vi "ProfilerTest.vi"() -> ()   [LabVIEW 2014] (continued)
"delVelocity"=0.0}, {"Time"=36.65000000000128, "delVelocity"=0.0}, {"Time"=36.660000000001276, "delVelocity"=0.0}, {"Time"=36.670000000001274, "delVelocity"=0.0}, {"Time"=36.68000000000127, "delVelocity"=0.0}, {"Time"=36.69000000000127, "delVelocity"=0.0}, {"Time"=36.70000000000127, "delVelocity"=0.0}, {"Time"=36.710000000001266, "delVelocity"=0.0}, {"Time"=36.720000000001264, "delVelocity"=0.0}, {"Time"=36.73000000000126, "delVelocity"=0.0}, {"Time"=36.74000000000126, "delVelocity"=0.0}, {"Time"=36.75000000000126, "delVelocity"=0.0}, {"Time"=36.760000000001256, "delVelocity"=0.0}, {"Time"=36.770000000001254, "delVelocity"=0.0}, {"Time"=36.78000000000125, "delVelocity"=0.0}, {"Time"=36.79000000000125, "delVelocity"=0.0}, {"Time"=36.80000000000125, "delVelocity"=0.0}, {"Time"=36.810000000001246, "delVelocity"=0.0}, {"Time"=36.820000000001244, "delVelocity"=0.0}, {"Time"=36.83000000000124, "delVelocity"=0.0}, {"Time"=36.84000000000124, "delVelocity"=0.0}, {"Time"=36.85000000000124, "delVelocity"=0.0}, {"Time"=36.860000000001236, "delVelocity"=0.0}, {"Time"=36.870000000001234, "delVelocity"=0.0}, {"Time"=36.88000000000123, "delVelocity"=0.0}, {"Time"=36.89000000000123, "delVelocity"=0.0}, {"Time"=36.90000000000123, "delVelocity"=0.0}, {"Time"=36.910000000001226, "delVelocity"=0.0}, {"Time"=36.920000000001224, "delVelocity"=0.0}, {"Time"=36.93000000000122, "delVelocity"=0.0}, {"Time"=36.94000000000122, "delVelocity"=0.0}, {"Time"=36.95000000000122, "delVelocity"=0.0}, {"Time"=36.960000000001216, "delVelocity"=0.0}, {"Time"=36.970000000001214, "delVelocity"=0.0}, {"Time"=36.98000000000121, "delVelocity"=0.0}, {"Time"=36.99000000000121, "delVelocity"=0.0}, {"Time"=37.00000000000121, "delVelocity"=0.0}, {"Time"=37.010000000001206, "delVelocity"=0.0}, {"Time"=37.020000000001204, "delVelocity"=0.0}, {"Time"=37.0300000000012, "delVelocity"=0.0}, {"Time"=37.0400000000012, "delVelocity"=0.0}, {"Time"=37.0500000000012, "delVelocity"=0.0}, {"Time"=37.060000000001196, "delVelocity"=0.0}, {"Time"=37.070000000001194, "delVelocity"=0.0}, {"Time"=37.08000000000119, "delVelocity"=0.0}, {"Time"=37.09000000000119, "delVelocity"=0.0}, {"Time"=37.10000000000119, "delVelocity"=0.0}, {"Time"=37.110000000001186, "delVelocity"=0.0}, {"Time"=37.120000000001184, "delVelocity"=0.0}, {"Time"=37.13000000000118, "delVelocity"=0.0}, {"Time"=37.14000000000118, "delVelocity"=0.0}, {"Time"=37.15000000000118, "delVelocity"=0.0}, {"Time"=37.160000000001176, "delVelocity"=0.0}, {"Time"=37.170000000001174, "delVelocity"=0.0}, {"Time"=37.18000000000117, "delVelocity"=0.0}, {"Time"=37.19000000000117, "delVelocity"=0.0}, {"Time"=37.20000000000117, "delVelocity"=0.0}, {"Time"=37.210000000001166, "delVelocity"=0.0}, {"Time"=37.220000000001164, "delVelocity"=0.0}, {"Time"=37.23000000000116, "delVelocity"=0.0}, {"Time"=37.24000000000116, "delVelocity"=0.0}, {"Time"=37.25000000000116, "delVelocity"=0.0}, {"Time"=37.260000000001156, "delVelocity"=0.0}, {"Time"=37.270000000001154, "delVelocity"=0.0}, {"Time"=37.28000000000115, "delVelocity"=0.0}, {"Time"=37.29000000000115, "delVelocity"=0.0}, {"Time"=37.30000000000115, "delVelocity"=0.0}, {"Time"=37.310000000001146, "delVelocity"=0.0}, {"Time"=37.320000000001144, "delVelocity"=0.0}, {"Time"=37.33000000000114, "delVelocity"=0.0}, {"Time"=37.34000000000114, "delVelocity"=0.0}, {"Time"=37.35000000000114, "delVelocity"=0.0}, {"Time"=37.360000000001136, "delVelocity"=0.0}, {"Time"=37.370000000001134, "delVelocity"=0.0}, {"Time"=37.38000000000113, "delVelocity"=0.0}, {"Time"=37.39000000000113, "delVelocity"=0.0}, {"Time"=37.40000000000113, "delVelocity"=0.0}, {"Time"=37.410000000001126, "delVelocity"=0.0}, {"Time"=37.420000000001124, "delVelocity"=0.0}, {"Time"=37.43000000000112, "delVelocity"=0.0}, {"Time"=37.44000000000112, "delVelocity"=0.0}, {"Time"=37.45000000000112, "delVelocity"=0.0}, {"Time"=37.460000000001116, "delVelocity"=0.0}, {"Time"=37.470000000001114, "delVelocity"=0.0}, {"Time"=37.48000000000111, "delVelocity"=0.0}, {"Time"=37.49000000000111, "delVelocity"=0.0}, {"Time"=37.50000000000111, "delVelocity"=0.0}, {"Time"=37.51000000000111, "delVelocity"=0.0}, {"Time"=37.520000000001104, "delVelocity"=0.0}, {"Time"=37.5300000000011, "delVelocity"=0.0}, {"Time"=37.5400000000011, "delVelocity"=0.0}, {"Time"=37.5500000000011, "delVelocity"=0.0}, {"Time"=37.5600000000011, "delVelocity"=0.0}, {"Time"=37.570000000001095, "delVelocity"=0.0}, {"Time"=37.58000000000109, "delVelocity"=0.0}, {"Time"=37.59000000000109, "delVelocity"=0.0}, {"Time"=37.60000000000109, "delVelocity"=0.0}, {"Time"=37.61000000000109, "delVelocity"=0.0}, {"Time"=37.620000000001085, "delVelocity"=0.0}, {"Time"=37.63000000000108, "delVelocity"=0.0}, {"Time"=37.64000000000108, "delVelocity"=0.0}, {"Time"=37.65000000000108, "delVelocity"=0.0}, {"Time"=37.66000000000108, "delVelocity"=0.0}, {"Time"=37.670000000001075, "delVelocity"=0.0}, {"Time"=37.68000000000107, "delVelocity"=0.0}, {"Time"=37.69000000000107, "delVelocity"=0.0}, {"Time"=37.70000000000107, "delVelocity"=0.0}, {"Time"=37.71000000000107, "delVelocity"=0.0}, {"Time"=37.720000000001065, "delVelocity"=0.0}, {"Time"=37.73000000000106, "delVelocity"=0.0}, {"Time"=37.74000000000106, "delVelocity"=0.0}, {"Time"=37.75000000000106, "delVelocity"=0.0}, {"Time"=37.76000000000106, "delVelocity"=0.0}, {"Time"=37.770000000001055, "delVelocity"=0.0}, {"Time"=37.78000000000105, "delVelocity"=0.0}, {"Time"=37.79000000000105, "delVelocity"=0.0}, {"Time"=37.80000000000105, "delVelocity"=0.0}, {"Time"=37.81000000000105, "delVelocity"=0.0}, {"Time"=37.820000000001045, "delVelocity"=0.0}, {"Time"=37.83000000000104, "delVelocity"=0.0}, {"Time"=37.84000000000104, "delVelocity"=0.0}, {"Time"=37.85000000000104, "delVelocity"=0.0}, {"Time"=37.86000000000104, "delVelocity"=0.0}, {"Time"=37.870000000001035, "delVelocity"=0.0}, {"Time"=37.88000000000103, "delVelocity"=0.0}, {"Time"=37.89000000000103, "delVelocity"=0.0}, {"Time"=37.90000000000103, "delVelocity"=0.0}, {"Time"=37.91000000000103, "delVelocity"=0.0}, {"Time"=37.920000000001025, "delVelocity"=0.0}, {"Time"=37.93000000000102, "delVelocity"=0.0}, {"Time"=37.94000000000102, "delVelocity"=0.0}, {"Time"=37.95000000000102, "delVelocity"=0.0}, {"Time"=37.96000000000102, "delVelocity"=0.0}, {"Time"=37.970000000001015, "delVelocity"=0.0}, {"Time"=37.98000000000101, "delVelocity"=0.0}, {"Time"=37.99000000000101, "delVelocity"=0.0}, {"Time"=38.00000000000101, "delVelocity"=0.0}, {"Time"=38.01000000000101, "delVelocity"=0.0}, {"Time"=38.020000000001005, "delVelocity"=0.0}, {"Time"=38.030000000001, "delVelocity"=0.0}, {"Time"=38.040000000001, "delVelocity"=0.0}, {"Time"=38.050000000001, "delVelocity"=0.0}, {"Time"=38.060000000001, "delVelocity"=0.0}, {"Time"=38.070000000000995, "delVelocity"=0.0}, {"Time"=38.08000000000099, "delVelocity"=0.0}, {"Time"=38.09000000000099, "delVelocity"=0.0}, {"Time"=38.10000000000099, "delVelocity"=0.0}, {"Time"=38.11000000000099, "delVelocity"=0.0}, {"Time"=38.120000000000985, "delVelocity"=0.0}, {"Time"=38.13000000000098, "delVelocity"=0.0}, {"Time"=38.14000000000098, "delVelocity"=0.0}, {"Time"=38.15000000000098, "delVelocity"=0.0}, {"Time"=38.16000000000098, "delVelocity"=0.0}, {"Time"=38.170000000000975, "delVelocity"=0.0}, {"Time"=38.18000000000097, "delVelocity"=0.0}, {"Time"=38.19000000000097, "delVelocity"=0.0}, {"Time"=38.20000000000097, "delVelocity"=0.0}, {"Time"=38.21000000000097, "delVelocity"=0.0}, {"Time"=38.220000000000965, "delVelocity"=0.0}, {"Time"=38.23000000000096, "delVelocity"=0.0}, {"Time"=38.24000000000096, "delVelocity"=0.0}, {"Time"=38.25000000000096, "delVelocity"=0.0}, {"Time"=38.26000000000096, "delVelocity"=0.0}, {"Time"=38.270000000000955, "delVelocity"=0.0}, {"Time"=38.28000000000095, "delVelocity"=0.0}, {"Time"=38.29000000000095, "delVelocity"=0.0}, {"Time"=38.30000000000095, "delVelocity"=0.0}, {"Time"=38.31000000000095, "delVelocity"=0.0}, {"Time"=38.320000000000945, "delVelocity"=0.0}, {"Time"=38.33000000000094, "delVelocity"=0.0}, {"Time"=38.34000000000094, "delVelocity"=0.0}, {"Time"=38.35000000000094, "delVelocity"=0.0}, {"Time"=38.36000000000094, "delVelocity"=0.0}, {"Time"=38.370000000000935, "delVelocity"=0.0}, {"Time"=38.38000000000093, "delVelocity"=0.0}, {"Time"=38.39000000000093, "delVelocity"=0.0}, {"Time"=38.40000000000093, "delVelocity"=0.0}, {"Time"=38.41000000000093, "delVelocity"=0.0}, {"Time"=38.420000000000925, "delVelocity"=0.0}, {"Time"=38.43000000000092, "delVelocity"=0.0}, {"Time"=38.44000000000092, "delVelocity"=0.0}, {"Time"=38.45000000000092, "delVelocity"=0.0}, {"Time"=38.46000000000092, "delVelocity"=0.0}, {"Time"=38.470000000000915, "delVelocity"=0.0}, {"Time"=38.48000000000091, "delVelocity"=0.0}, {"Time"=38.49000000000091, "delVelocity"=0.0}, {"Time"=38.50000000000091, "delVelocity"=0.0}, {"Time"=38.51000000000091, "delVelocity"=0.0}, {"Time"=38.520000000000906, "delVelocity"=0.0}, {"Time"=38.5300000000009, "delVelocity"=0.0}, {"Time"=38.5400000000009, "delVelocity"=0.0}, {"Time"=38.5500000000009, "delVelocity"=0.0}, {"Time"=38.5600000000009, "delVelocity"=0.0}, {"Time"=38.570000000000896, "delVelocity"=0.0}, {"Time"=38.580000000000894, "delVelocity"=0.0}, {"Time"=38.59000000000089, "delVelocity"=0.0}, {"Time"=38.60000000000089, "delVelocity"=0.0}, {"Time"=38.61000000000089, "delVelocity"=0.0}, {"Time"=38.620000000000886, "delVelocity"=0.0}, {"Time"=38.630000000000884, "delVelocity"=0.0}, {"Time"=38.64000000000088, "delVelocity"=0.0}, {"Time"=38.65000000000088, "delVelocity"=0.0}, {"Time"=38.66000000000088, "delVelocity"=0.0}, {"Time"=38.670000000000876, "delVelocity"=0.0}, {"Time"=38.680000000000874, "delVelocity"=0.0}, {"Time"=38.69000000000087, "delVelocity"=0.0}, {"Time"=38.70000000000087, "delVelocity"=0.0}, {"Time"=38.71000000000087, "delVelocity"=0.0}, {"Time"=38.720000000000866, "delVelocity"=0.0}, {"Time"=38.730000000000864, "delVelocity"=0.0}, {"Time"=38.74000000000086, "delVelocity"=0.0}, {"Time"=38.75000000000086, "delVelocity"=0.0}, {"Time"=38.76000000000086, "delVelocity"=0.0}, {"Time"=38.770000000000856, "delVelocity"=0.0}, {"Time"=38.780000000000854, "delVelocity"=0.0}, {"Time"=38.79000000000085, "delVelocity"=0.0}, {"Time"=38.80000000000085, "delVelocity"=0.0}, {"Time"=38.81000000000085, "delVelocity"=0.0}, {"Time"=38.820000000000846, "delVelocity"=0.0}, {"Time"=38.830000000000844, "delVelocity"=0.0}, {"Time"=38.84000000000084, "delVelocity"=0.0}, {"Time"=38.85000000000084, "delVelocity"=0.0}, {"Time"=38.86000000000084, "delVelocity"=0.0}, {"Time"=38.870000000000836, "delVelocity"=0.0}, {"Time"=38.880000000000834, "delVelocity"=0.0}, {"Time"=38.89000000000083, "delVelocity"=0.0}, {"Time"=38.90000000000083, "delVelocity"=0.0}, {"Time"=38.91000000000083, "delVelocity"=0.0}, {"Time"=38.920000000000826, "delVelocity"=0.0}, {"Time"=38.930000000000824, "delVelocity"=0.0}, {"Time"=38.94000000000082, "delVelocity"=0.0}, {"Time"=38.95000000000082, "delVelocity"=0.0}, {"Time"=38.96000000000082, "delVelocity"=0.0}, {"Time"=38.970000000000816, "delVelocity"=0.0}, {"Time"=38.980000000000814, "delVelocity"=0.0}, {"Time"=38.99000000000081, "delVelocity"=0.0}, {"Time"=39.00000000000081, "delVelocity"=0.0}, {"Time"=39.01000000000081, "delVelocity"=0.0}, {"Time"=39.020000000000806, "delVelocity"=0.0}, {"Time"=39.030000000000804, "delVelocity"=0.0}, {"Time"=39.0400000000008, "delVelocity"=0.0}, {"Time"=39.0500000000008, "delVelocity"=0.0}, {"Time"=39.0600000000008, "delVelocity"=0.0}, {"Time"=39.070000000000796, "delVelocity"=0.0}, {"Time"=39.080000000000794, "delVelocity"=0.0}, {"Time"=39.09000000000079, "delVelocity"=0.0}, {"Time"=39.10000000000079, "delVelocity"=0.0}, {"Time"=39.11000000000079, "delVelocity"=0.0}, {"Time"=39.120000000000786, "delVelocity"=0.0}, {"Time"=39.130000000000784, "delVelocity"=0.0}, {"Time"=39.14000000000078, "delVelocity"=0.0}, {"Time"=39.15000000000078, "delVelocity"=0.0}, {"Time"=39.16000000000078, "delVelocity"=0.0}, {"Time"=39.170000000000776, "delVelocity"=0.0}, {"Time"=39.180000000000774, "delVelocity"=0.0}, {"Time"=39.19000000000077, "delVelocity"=0.0}, {"Time"=39.20000000000077, "delVelocity"=0.0}, {"Time"=39.21000000000077, "delVelocity"=0.0}, {"Time"=39.220000000000766, "delVelocity"=0.0}, {"Time"=39.230000000000764, "delVelocity"=0.0}, {"Time"=39.24000000000076, "delVelocity"=0.0}, {"Time"=39.25000000000076, "delVelocity"=0.0}, {"Time"=39.26000000000076, "delVelocity"=0.0}, {"Time"=39.270000000000756, "delVelocity"=0.0}, {"Time"=39.280000000000754, "delVelocity"=0.0}, {"Time"=39.29000000000075, "delVelocity"=0.0}, {"Time"=39.30000000000075, "delVelocity"=0.0}, {"Time"=39.31000000000075, "delVelocity"=0.0}, {"Time"=39.320000000000746, "delVelocity"=0.0}, {"Time"=39.330000000000744, "delVelocity"=0.0}, {"Time"=39.34000000000074, "delVelocity"=0.0}, {"Time"=39.35000000000074, "delVelocity"=0.0}, {"Time"=39.36000000000074, "delVelocity"=0.0}, {"Time"=39.370000000000736, "delVelocity"=0.0}, {"Time"=39.380000000000734, "delVelocity"=0.0}, {"Time"=39.39000000000073, "delVelocity"=0.0}, {"Time"=39.40000000000073, "delVelocity"=0.0}, {"Time"=39.41000000000073, "delVelocity"=0.0}, {"Time"=39.42000000000073, "delVelocity"=0.0}, {"Time"=39.430000000000724, "delVelocity"=0.0}, {"Time"=39.44000000000072, "delVelocity"=0.0}, {"Time"=39.45000000000072, "delVelocity"=0.0}, {"Time"=39.46000000000072, "delVelocity"=0.0}, {"Time"=39.47000000000072, "delVelocity"=0.0}, {"Time"=39.480000000000715, "delVelocity"=0.0}, {"Time"=39.49000000000071, "delVelocity"=0.0}, {"Time"=39.50000000000071, "delVelocity"=0.0}, {"Time"=39.51000000000071, "delVelocity"=0.0}, {"Time"=39.52000000000071, "delVelocity"=0.0}, {"Time"=39.530000000000705, "delVelocity"=0.0}, {"Time"=39.5400000000007, "delVelocity"=0.0}, {"Time"=39.5500000000007, "delVelocity"=0.0}, {"Time"=39.5600000000007, "delVelocity"=0.0}, {"Time"=39.5700000000007, "delVelocity"=0.0}, {"Time"=39.580000000000695, "delVelocity"=0.0}, {"Time"=39.59000000000069, "delVelocity"=0.0}, {"Time"=39.60000000000069, "delVelocity"=0.0}, {"Time"=39.61000000000069, "delVelocity"=0.0}, {"Time"=39.62000000000069, "delVelocity"=0.0}, {"Time"=39.630000000000685, "delVelocity"=0.0}, {"Time"=39.64000000000068, "delVelocity"=0.0}, {"Time"=39.65000000000068, "delVelocity"=0.0}, {"Time"=39.66000000000068, "delVelocity"=0.0}, {"Time"=39.67000000000068, "delVelocity"=0.0}, {"Time"=39.680000000000675, "delVelocity"=0.0}, {"Time"=39.69000000000067, "delVelocity"=0.0}, {"Time"=39.70000000000067, "delVelocity"=0.0}, {"Time"=39.71000000000067, "delVelocity"=0.0}, {"Time"=39.72000000000067, "delVelocity"=0.0}, {"Time"=39.730000000000665, "delVelocity"=0.0}, {"Time"=39.74000000000066, "delVelocity"=0.0}, {"Time"=39.75000000000066, "delVelocity"=0.0}, {"Time"=39.76000000000066, "delVelocity"=0.0}, {"Time"=39.77000000000066, "delVelocity"=0.0}, {"Time"=39.780000000000655, "delVelocity"=0.0}, {"Time"=39.79000000000065, "delVelocity"=0.0}, {"Time"=39.80000000000065, "delVelocity"=0.0}, {"Time"=39.81000000000065, "delVelocity"=0.0}, {"Time"=39.82000000000065, "delVelocity"=0.0}, {"Time"=39.830000000000645, "delVelocity"=0.0}, {"Time"=39.84000000000064, "delVelocity"=0.0}, {"Time"=39.85000000000064, "delVelocity"=0.0}, {"Time"=39.86000000000064, "delVelocity"=0.0}, {"Time"=39.87000000000064, "delVelocity"=0.0}, {"Time"=39.880000000000635, "delVelocity"=0.0}, {"Time"=39.89000000000063, "delVelocity"=0.0}, {"Time"=39.90000000000063, "delVelocity"=0.0}, {"Time"=39.91000000000063, "delVelocity"=0.0}, {"Time"=39.92000000000063, "delVelocity"=0.0}, {"Time"=39.930000000000625, "delVelocity"=0.0}, {"Time"=39.94000000000062, "delVelocity"=0.0}, {"Time"=39.95000000000062, "delVelocity"=0.0}, {"Time"=39.96000000000062, "delVelocity"=0.0}, {"Time"=39.97000000000062, "delVelocity"=0.0}, {"Time"=39.980000000000615, "delVelocity"=0.0}, {"Time"=39.99000000000061, "delVelocity"=0.0}, {"Time"=0.0, "delVelocity"=0.0}]}, ...(4 in all)]
  out "yAccel":T4(array[cluster])=[{"A"=5.0, "B"=7.853981633974483, "Start"=-0.2, "End"=0.2, "Center"=0.0, "Velocity"=0.0, "Position"=0.0}, {"A"=-3.0533720235915274, "B"=16.375338351724178, "Start"=0.4040754888200826, "End"=0.5959245111799174, "Center"=0.5, "Velocity"=1.0, "Position"=0.4040754888200826}, {"A"=-5.0, "B"=5.553603672697958, "Start"=0.9242640687119285, "End"=1.4899494936611664, "Center"=1.2071067811865475, "Velocity"=0.7071067811865475, "Position"=0.8}, {"A"=0.0, "B"=0.0, "Start"=1.914213562373095, "End"=1.914213562373095, "Center"=1.914213562373095, "Velocity"=-0.7071067811865475, "Position"=0.5}, {"A"=5.0, "B"=5.553603672697958, "Start"=2.3384776310850235, "End"=2.9041630560342613, "Center"=2.6213203435596424, "Velocity"=-0.7071067811865475, "Position"=0.19999999999999998}, {"A"=-5.0, "B"=4.60075592255305, "Start"=2.9870057685088804, "End"=3.6698484809834993, "Center"=3.32842712474619, "Velocity"=0.7071067811865475, "Position"=0.2585786437626905}, {"A"=0.0, "B"=0.0, "Start"=3.82842712474619, "End"=3.82842712474619, "Center"=3.82842712474619, "Velocity"=-1.0, "Position"=0.0}]
  out "xAccel":T4(array[cluster])=[{"A"=0.0, "B"=0.0, "Start"=0.0, "End"=0.0, "Center"=0.0, "Velocity"=0.0, "Position"=0.0}, {"A"=4.7442499832879435, "B"=10.539073652554059, "Start"=0.35095499105709094, "End"=0.6490450089429091, "Center"=0.5, "Velocity"=0.0, "Position"=0.0}, {"A"=0.0, "B"=0.0, "Start"=1.2071067811865475, "End"=1.2071067811865475, "Center"=1.2071067811865475, "Velocity"=0.7071067811865475, "Position"=0.5}, {"A"=-5.0, "B"=5.553603672697958, "Start"=1.631370849898476, "End"=2.197056274847714, "Center"=1.914213562373095, "Velocity"=0.7071067811865475, "Position"=0.8}, {"A"=0.0, "B"=0.0, "Start"=2.6213203435596424, "End"=2.6213203435596424, "Center"=2.6213203435596424, "Velocity"=-0.7071067811865475, "Position"=0.5}, {"A"=4.7442499832879435, "B"=10.539073652554059, "Start"=3.1793821158032807, "End"=3.477472133689099, "Center"=3.32842712474619, "Velocity"=-0.7071067811865475, "Position"=0.10539073652554058}, {"A"=0.0, "B"=0.0, "Start"=3.82842712474619, "End"=3.82842712474619, "Center"=3.82842712474619, "Velocity"=0.0, "Position"=0.0}]
  out "Accel":cluster{cluster{"Time":dbl, "Velocity":dbl}[]}[](graph)=[{[{"Time"=0.0, "Velocity"=0.0}, {"Time"=0.0, "Velocity"=0.0}, {"Time"=0.0, "Velocity"=0.0}, {"Time"=0.0, "Velocity"=0.0}, {"Time"=0.0, "Velocity"=0.0}, {"Time"=0.0, "Velocity"=0.0}, {"Time"=0.0, "Velocity"=0.0}, {"Time"=0.0, "Velocity"=0.0}, {"Time"=0.0, "Velocity"=0.0}, {"Time"=0.0, "Velocity"=0.0}, {"Time"=0.0, "Velocity"=0.0}, {"Time"=0.0, "Velocity"=0.0}, {"Time"=0.0, "Velocity"=0.0}, {"Time"=0.0, "Velocity"=0.0}, {"Time"=0.0, "Velocity"=0.0}, {"Time"=0.0, "Velocity"=0.0}, {"Time"=0.0, "Velocity"=0.0}, {"Time"=0.0, "Velocity"=0.0}, {"Time"=0.0, "Velocity"=0.0}, {"Time"=0.0, "Velocity"=0.0}, {"Time"=0.0, "Velocity"=0.0}, {"Time"=0.0, "Velocity"=0.0}, {"Time"=0.0, "Velocity"=0.0}, {"Time"=0.0, "Velocity"=0.0}, {"Time"=0.0, "Velocity"=0.0}, {"Time"=0.0, "Velocity"=0.0}, {"Time"=0.0, "Velocity"=0.0}, {"Time"=0.0, "Velocity"=0.0}, {"Time"=0.0, "Velocity"=0.0}, {"Time"=0.0, "Velocity"=0.0}, {"Time"=0.0, "Velocity"=0.0}, {"Time"=0.0, "Velocity"=0.0}, {"Time"=0.0, "Velocity"=0.0}, {"Time"=0.0, "Velocity"=0.0}, {"Time"=0.0, "Velocity"=0.0}, {"Time"=0.0, "Velocity"=0.0}, {"Time"=0.0, "Velocity"=0.0}, {"Time"=0.0, "Velocity"=0.0}, {"Time"=0.0, "Velocity"=0.0}, {"Time"=0.0, "Velocity"=0.0}, {"Time"=0.0, "Velocity"=0.0}, {"Time"=0.0, "Velocity"=0.0}, {"Time"=0.0, "Velocity"=0.0}, {"Time"=0.0, "Velocity"=0.0}, {"Time"=0.0, "Velocity"=0.0}, {"Time"=0.0, "Velocity"=0.0}, {"Time"=0.0, "Velocity"=0.0}, {"Time"=0.0, "Velocity"=0.0}, {"Time"=0.0, "Velocity"=0.0}, {"Time"=0.0, "Velocity"=0.0}, {"Time"=0.0, "Velocity"=0.0}, {"Time"=0.0, "Velocity"=0.0}, {"Time"=0.0, "Velocity"=0.0}, {"Time"=0.0, "Velocity"=0.0}, {"Time"=0.0, "Velocity"=0.0}, {"Time"=0.0, "Velocity"=0.0}, {"Time"=0.0, "Velocity"=0.0}, {"Time"=0.0, "Velocity"=0.0}, {"Time"=0.0, "Velocity"=0.0}, {"Time"=0.0, "Velocity"=0.0}, {"Time"=0.0, "Velocity"=0.0}, {"Time"=0.0, "Velocity"=0.0}, {"Time"=0.0, "Velocity"=0.0}, {"Time"=0.0, "Velocity"=0.0}, {"Time"=0.0, "Velocity"=0.0}, {"Time"=0.0, "Velocity"=0.0}, {"Time"=0.0, "Velocity"=0.0}, {"Time"=0.0, "Velocity"=0.0}, {"Time"=0.0, "Velocity"=0.0}, {"Time"=0.0, "Velocity"=0.0}, {"Time"=0.0, "Velocity"=0.0}, {"Time"=0.0, "Velocity"=0.0}, {"Time"=0.0, "Velocity"=0.0}, {"Time"=0.0, "Velocity"=0.0}, {"Time"=0.0, "Velocity"=0.0}, {"Time"=0.0, "Velocity"=0.0}, {"Time"=0.0, "Velocity"=0.0}, {"Time"=0.0, "Velocity"=0.0}, {"Time"=0.0, "Velocity"=0.0}, {"Time"=0.0, "Velocity"=0.0}, {"Time"=0.0, "Velocity"=0.0}, {"Time"=0.0, "Velocity"=0.0}, {"Time"=0.0, "Velocity"=0.0}, {"Time"=0.0, "Velocity"=0.0}, {"Time"=0.0, "Velocity"=0.0}, {"Time"=0.0, "Velocity"=0.0}, {"Time"=0.0, "Velocity"=0.0}, {"Time"=0.0, "Velocity"=0.0}, {"Time"=0.0, "Velocity"=0.0}, {"Time"=0.0, "Velocity"=0.0}, {"Time"=0.0, "Velocity"=0.0}, {"Time"=0.0, "Velocity"=0.0}, {"Time"=0.0, "Velocity"=0.0}, {"Time"=0.0, "Velocity"=0.0}, {"Time"=0.0, "Velocity"=0.0}, {"Time"=0.0, "Velocity"=0.0}, {"Time"=0.0, "Velocity"=0.0}, {"Time"=0.0, "Velocity"=0.0}, {"Time"=0.0, "Velocity"=0.0}, {"Time"=0.0, "Velocity"=0.0}, {"Time"=0.0, "Velocity"=0.0}, {"Time"=0.35095531925568213, "Velocity"=5.50736024568391e-11}, {"Time"=0.3539359458930411, "Velocity"=0.004681003307826736}, {"Time"=0.3569169329724022, "Velocity"=0.018705771687410763}, {"Time"=0.3598980439615304, "Velocity"=0.04202011351167813}, {"Time"=0.3628788161034107, "Velocity"=0.07452740216306052}, {"Time"=0.3658595272222378, "Velocity"=0.11610053792080005}, {"Time"=0.3688406611141025, "Velocity"=0.16658382483664627}, {"Time"=0.3718215316238896, "Velocity"=0.2257671329984986}, {"Time"=0.37480228037519364, "Velocity"=0.29341803418359613}, {"Time"=0.3777830973771714, "Velocity"=0.3692736379683199}, {"Time"=0.380764072133267, "Velocity"=0.4530377768984485}, {"Time"=0.3837451854232035, "Velocity"=0.5443804709605526}, {"Time"=0.38672614678717, "Velocity"=0.642932269145972}, {"Time"=0.3897067735390129, "Velocity"=0.7482964854099229}, {"Time"=0.39268779230328543, "Velocity"=0.8600831387079992}, {"Time"=0.3956686493693256, "Velocity"=0.9778310646207633}, {"Time"=0.39864961030082646, "Velocity"=1.1010858577858063}, {"Time"=0.40163042391800347, "Velocity"=1.2293506118536994}, {"Time"=0.40461134537834614, "Velocity"=1.3621299917800744}, {"Time"=0.40759213500004476, "Velocity"=1.498889288710395}, {"Time"=0.4105733396656944, "Velocity"=1.6391143292638135}, {"Time"=0.4135539403558606, "Velocity"=1.7822035689878706}, {"Time"=0.4165348905749282, "Velocity"=1.9276376584907495}, {"Time"=0.41951578640723575, "Velocity"=2.0748232975591545}, {"Time"=0.42249679151073805, "Velocity"=2.223187700059486}, {"Time"=0.4254776474532113, "Velocity"=2.3721324733928784}, {"Time"=0.42845858580727364, "Velocity"=2.5210813296808565}, {"Time"=0.4314396484569505, "Velocity"=2.66944847406714}, {"Time"=0.4344202596314551, "Velocity"=2.816619916696366}, {"Time"=0.43740137519387107, "Velocity"=2.9620619079454316}, {"Time"=0.4403821725508091, "Velocity"=3.105160219697094}, {"Time"=0.44336302583933573, "Velocity"=3.245368375837273}, {"Time"=0.44634387547325305, "Velocity"=3.3821301821391057}, {"Time"=0.4493247970269584, "Velocity"=3.514909245469887}, {"Time"=0.45230571043094475, "Velocity"=3.6431778524652842}, {"Time"=0.4552867137489194, "Velocity"=3.766433786802063}, {"Time"=0.4582676835999003, "Velocity"=3.884185350994328}, {"Time"=0.46124842978267827, "Velocity"=3.99596107220399}, {"Time"=0.4642292839309622, "Velocity"=4.101332611153013}, {"Time"=0.46721035372627223, "Velocity"=4.199886840806099}, {"Time"=0.47019116678105355, "Velocity"=4.291219363025584}, {"Time"=0.47317195740077206, "Velocity"=4.37497793755458}, {"Time"=0.47615286456958295, "Velocity"=4.450835554257804}, {"Time"=0.479134006270323, "Velocity"=4.518494403973455}, {"Time"=0.48211476749612264, "Velocity"=4.577674138445382}, {"Time"=0.4850958093220748, "Velocity"=4.628154724183214}, {"Time"=0.48807652197732365, "Velocity"=4.669726851819185}, {"Time"=0.4910574291962836, "Velocity"=4.702234357339671}, {"Time"=0.4940382028607463, "Velocity"=4.725545104792937}, {"Time"=0.49701922558438005, "Velocity"=4.739569547693048}, {"Time"=0.5000002690275388, "Velocity"=4.744249999961862}, {"Time"=0.5029810686846331, "Velocity"=4.739568623821157}, {"Time"=0.5059620123716997, "Velocity"=4.725543755980428}, {"Time"=0.5089429652918902, "Velocity"=4.702230661326216}, {"Time"=0.5119236749950736, "Velocity"=4.669724402571721}, {"Time"=0.5149047704873164, "Velocity"=4.628145765646637}, {"Time"=0.5178856707272734, "Velocity"=4.577666072383549}, {"Time"=0.520866503859561, "Velocity"=4.518483543861212}, {"Time"=0.523847516316558, "Velocity"=4.450826379548527}, {"Time"=0.5268283322097902, "Velocity"=4.374970178476992}, {"Time"=0.5298090653014678, "Velocity"=4.291212542301367}, {"Time"=0.5327901478802014, "Velocity"=4.199870854007082}, {"Time"=0.5357708251342688, "Velocity"=4.101328878141011}, {"Time"=0.5387519365752801, "Velocity"=3.9959477190167645}, {"Time"=0.5417326532258172, "Velocity"=3.8841723745863823}, {"Time"=0.5447136608295621, "Velocity"=3.766418634790069}, {"Time"=0.5476947464554902, "Velocity"=3.6431585643356734}, {"Time"=0.5506753637730458, "Velocity"=3.514902199965208}, {"Time"=0.5536565483461207, "Velocity"=3.3821110079509995}, {"Time"=0.5566371342578786, "Velocity"=3.245360933108672}, {"Time"=0.5596181273960594, "Velocity"=3.1051459563777444}, {"Time"=0.5625990777602468, "Velocity"=2.9620399717640513}, {"Time"=0.5655800049566987, "Velocity"=2.8166069216136798}, {"Time"=0.568560732875166, "Velocity"=2.6694295578145515}, {"Time"=0.5715419247218683, "Velocity"=2.5210558535911827}, {"Time"=0.5745228056007107, "Velocity"=2.372109820695952}, {"Time"=0.5775037267700815, "Velocity"=2.223161837155251}, {"Time"=0.5804844515939579, "Velocity"=2.074811491335522}, {"Time"=0.5834654466221451, "Velocity"=1.9276210972758885}, {"Time"=0.5864463583362974, "Velocity"=1.782189103585959}, {"Time"=0.5894270243328484, "Velocity"=1.6390970200848998}, {"Time"=0.5924082186970084, "Velocity"=1.4988728457687575}, {"Time"=0.5953890228973194, "Velocity"=1.3621133304961972}, {"Time"=0.5983700078816026, "Velocity"=1.2293316924286313}, {"Time"=0.6013507854827487, "Velocity"=1.1010691492255635}, {"Time"=0.6043318079934541, "Velocity"=0.9778125639286918}, {"Time"=0.6073124405489622, "Velocity"=0.8600741679083297}, {"Time"=0.6102933319138173, "Velocity"=0.7482926418177279}, {"Time"=0.6132743316865582, "Velocity"=0.6429158922144192}, {"Time"=0.6162551894170679, "Velocity"=0.5443685243202626}, {"Time"=0.6192361682993021, "Velocity"=0.45303071077147344}, {"Time"=0.6222172382105677, "Velocity"=0.36926464717276025}, {"Time"=0.6251978283531981, "Velocity"=0.29341541516543757}, {"Time"=0.6281787093500688, "Velocity"=0.22576200288591172}, {"Time"=0.6311599266610616, "Velocity"=0.1665730061296175}, {"Time"=0.6341408500489021, "Velocity"=0.116094708820569}, {"Time"=0.6371216254044041, "Velocity"=0.07452191223685314}, {"Time"=0.6401025565856091, "Velocity"=0.042014486916333305}, {"Time"=0.6430832903776259, "Velocity"=0.0187043720224209}, {"Time"=0.6460641319394195, "Velocity"=0.004680758949891532}, {"Time"=0.6490452493606549, "Velocity"=3.1716017876300603e-11}, {"Time"=1.2071067811865475, "Velocity"=0.0}, {"Time"=1.2071067811865475, "Velocity"=0.0}, {"Time"=1.2071067811865475, "Velocity"=0.0}, {"Time"=1.2071067811865475, "Velocity"=0.0}, {"Time"=1.2071067811865475, "Velocity"=0.0}, {"Time"=1.2071067811865475, "Velocity"=0.0}, {"Time"=1.2071067811865475, "Velocity"=0.0}, {"Time"=1.2071067811865475, "Velocity"=0.0}, {"Time"=1.2071067811865475, "Velocity"=0.0}, {"Time"=1.2071067811865475, "Velocity"=0.0}, {"Time"=1.2071067811865475, "Velocity"=0.0}, {"Time"=1.2071067811865475, "Velocity"=0.0}, {"Time"=1.2071067811865475, "Velocity"=0.0}, {"Time"=1.2071067811865475, "Velocity"=0.0}, {"Time"=1.2071067811865475, "Velocity"=0.0}, {"Time"=1.2071067811865475, "Velocity"=0.0}, {"Time"=1.2071067811865475, "Velocity"=0.0}, {"Time"=1.2071067811865475, "Velocity"=0.0}, {"Time"=1.2071067811865475, "Velocity"=0.0}, {"Time"=1.2071067811865475, "Velocity"=0.0}, {"Time"=1.2071067811865475, "Velocity"=0.0}, {"Time"=1.2071067811865475, "Velocity"=0.0}, {"Time"=1.2071067811865475, "Velocity"=0.0}, {"Time"=1.2071067811865475, "Velocity"=0.0}, {"Time"=1.2071067811865475, "Velocity"=0.0}, {"Time"=1.2071067811865475, "Velocity"=0.0}, {"Time"=1.2071067811865475, "Velocity"=0.0}, {"Time"=1.2071067811865475, "Velocity"=0.0}, {"Time"=1.2071067811865475, "Velocity"=0.0}, {"Time"=1.2071067811865475, "Velocity"=0.0}, {"Time"=1.2071067811865475, "Velocity"=0.0}, {"Time"=1.2071067811865475, "Velocity"=0.0}, {"Time"=1.2071067811865475, "Velocity"=0.0}, {"Time"=1.2071067811865475, "Velocity"=0.0}, {"Time"=1.2071067811865475, "Velocity"=0.0}, {"Time"=1.2071067811865475, "Velocity"=0.0}, {"Time"=1.2071067811865475, "Velocity"=0.0}, {"Time"=1.2071067811865475, "Velocity"=0.0}, {"Time"=1.2071067811865475, "Velocity"=0.0}, {"Time"=1.2071067811865475, "Velocity"=0.0}, {"Time"=1.2071067811865475, "Velocity"=0.0}, {"Time"=1.2071067811865475, "Velocity"=0.0}, {"Time"=1.2071067811865475, "Velocity"=0.0}, {"Time"=1.2071067811865475, "Velocity"=0.0}, {"Time"=1.2071067811865475, "Velocity"=0.0}, {"Time"=1.2071067811865475, "Velocity"=0.0}, {"Time"=1.2071067811865475, "Velocity"=0.0}, {"Time"=1.2071067811865475, "Velocity"=0.0}, {"Time"=1.2071067811865475, "Velocity"=0.0}, {"Time"=1.2071067811865475, "Velocity"=0.0}, {"Time"=1.2071067811865475, "Velocity"=0.0}, {"Time"=1.2071067811865475, "Velocity"=0.0}, {"Time"=1.2071067811865475, "Velocity"=0.0}, {"Time"=1.2071067811865475, "Velocity"=0.0}, {"Time"=1.2071067811865475, "Velocity"=0.0}, {"Time"=1.2071067811865475, "Velocity"=0.0}, {"Time"=1.2071067811865475, "Velocity"=0.0}, {"Time"=1.2071067811865475, "Velocity"=0.0}, {"Time"=1.2071067811865475, "Velocity"=0.0}, {"Time"=1.2071067811865475, "Velocity"=0.0}, {"Time"=1.2071067811865475, "Velocity"=0.0}, {"Time"=1.2071067811865475, "Velocity"=0.0}, {"Time"=1.2071067811865475, "Velocity"=0.0}, {"Time"=1.2071067811865475, "Velocity"=0.0}, {"Time"=1.2071067811865475, "Velocity"=0.0}, {"Time"=1.2071067811865475, "Velocity"=0.0}, {"Time"=1.2071067811865475, "Velocity"=0.0}, {"Time"=1.2071067811865475, "Velocity"=0.0}, {"Time"=1.2071067811865475, "Velocity"=0.0}, {"Time"=1.2071067811865475, "Velocity"=0.0}, {"Time"=1.2071067811865475, "Velocity"=0.0}, {"Time"=1.2071067811865475, "Velocity"=0.0}, {"Time"=1.2071067811865475, "Velocity"=0.0}, {"Time"=1.2071067811865475, "Velocity"=0.0}, {"Time"=1.2071067811865475, "Velocity"=0.0}, {"Time"=1.2071067811865475, "Velocity"=0.0}, {"Time"=1.2071067811865475, "Velocity"=0.0}, {"Time"=1.2071067811865475, "Velocity"=0.0}, {"Time"=1.2071067811865475, "Velocity"=0.0}, {"Time"=1.2071067811865475, "Velocity"=0.0}, {"Time"=1.2071067811865475, "Velocity"=0.0}, {"Time"=1.2071067811865475, "Velocity"=0.0}, {"Time"=1.2071067811865475, "Velocity"=0.0}, {"Time"=1.2071067811865475, "Velocity"=0.0}, {"Time"=1.2071067811865475, "Velocity"=0.0}, {"Time"=1.2071067811865475, "Velocity"=0.0}, {"Time"=1.2071067811865475, "Velocity"=0.0}, {"Time"=1.2071067811865475, "Velocity"=0.0}, {"Time"=1.2071067811865475, "Velocity"=0.0}, {"Time"=1.2071067811865475, "Velocity"=0.0}, {"Time"=1.2071067811865475, "Velocity"=0.0}, {"Time"=1.2071067811865475, "Velocity"=0.0}, {"Time"=1.2071067811865475, "Velocity"=0.0}, {"Time"=1.2071067811865475, "Velocity"=0.0}, {"Time"=1.2071067811865475, "Velocity"=0.0}, {"Time"=1.2071067811865475, "Velocity"=0.0}, {"Time"=1.2071067811865475, "Velocity"=0.0}, {"Time"=1.2071067811865475, "Velocity"=0.0}, {"Time"=1.2071067811865475, "Velocity"=0.0}, {"Time"=1.2071067811865475, "Velocity"=0.0}, {"Time"=1.2071067811865475, "Velocity"=0.0}, {"Time"=1.6313709713857558, "Velocity"=-1.7080866399157617e-11}, {"Time"=1.6370282709806934, "Velocity"=-0.004933375727589114}, {"Time"=1.6426849079991253, "Velocity"=-0.019712884672038487}, {"Time"=1.6483415996983244, "Velocity"=-0.044280487862295104}, {"Time"=1.6539986753458422, "Velocity"=-0.07854178978642275}, {"Time"=1.6596556901806123, "Velocity"=-0.12235970811397348}, {"Time"=1.665312360236421, "Velocity"=-0.1755580957494901}, {"Time"=1.6709691529406534, "Velocity"=-0.23793084760329003}, {"Time"=1.676626212913127, "Velocity"=-0.30923433515789267}, {"Time"=1.6822827123498711, "Velocity"=-0.3891760634774344}, {"Time"=1.6879400617709552, "Velocity"=-0.47746107896069007}, {"Time"=1.6935962842751575, "Velocity"=-0.5737095830376884}, {"Time"=1.6992532063435852, "Velocity"=-0.6775718764786762}, {"Time"=1.7049105370471096, "Velocity"=-0.7886349059724539}, {"Time"=1.7105672640182004, "Velocity"=-0.9064401325634146}, {"Time"=1.7162236979713061, "Velocity"=-1.0305275471784532}, {"Time"=1.721880645195221, "Velocity"=-1.160425471206782}, {"Time"=1.7275375756120264, "Velocity"=-1.295609849283178}, {"Time"=1.733194266958434, "Velocity"=-1.4355415268732759}, {"Time"=1.7388511806477678, "Velocity"=-1.5796796348273192}, {"Time"=1.7445084006521792, "Velocity"=-1.7274579929979808}, {"Time"=1.7501651906164457, "Velocity"=-1.8782740498239738}, {"Time"=1.7558218830375498, "Velocity"=-2.031541058872726}, {"Time"=1.7614790199438888, "Velocity"=-2.1866690009673215}, {"Time"=1.7671359216104991, "Velocity"=-2.343027121799203}, {"Time"=1.7727927595404411, "Velocity"=-2.5000029834813993}, {"Time"=1.7784496560344534, "Velocity"=-2.6569804563884114}, {"Time"=1.7841064035118543, "Velocity"=-2.8133342845614884}, {"Time"=1.7897631395459257, "Velocity"=-2.9684512598511636}, {"Time"=1.7954199999975988, "Velocity"=-3.1217228953509206}, {"Time"=1.8010768994328874, "Velocity"=-3.272541898469922}, {"Time"=1.806733605263529, "Velocity"=-3.4203069841090854}, {"Time"=1.8123907523050318, "Velocity"=-3.5644513141656216}, {"Time"=1.818047178727535, "Velocity"=-3.7043767709226803}, {"Time"=1.8237041515421901, "Velocity"=-3.83956263130222}, {"Time"=1.8293612186562676, "Velocity"=-3.969463746218262}, {"Time"=1.8350181774083052, "Velocity"=-4.093562803594636}, {"Time"=1.8406747486420618, "Velocity"=-4.211364719437065}, {"Time"=1.8463318125129005, "Velocity"=-4.322422699677098}, {"Time"=1.851988715518848, "Velocity"=-4.4262850290876035}, {"Time"=1.8576453562736979, "Velocity"=-4.522540779260416}, {"Time"=1.8633022020871002, "Velocity"=-4.610818137383916}, {"Time"=1.8689592132708241, "Velocity"=-4.690767296734542}, {"Time"=1.8746157273145294, "Velocity"=-4.762064140129214}, {"Time"=1.8802727897096965, "Velocity"=-4.824440327506827}, {"Time"=1.8859296217848325, "Velocity"=-4.877640358565102}, {"Time"=1.8915865989596123, "Velocity"=-4.921458003809648}, {"Time"=1.8972436635459324, "Velocity"=-4.955719299066888}, {"Time"=1.9029002654742275, "Velocity"=-4.980286660385663}, {"Time"=1.9085572145244145, "Velocity"=-4.995066940400685}, {"Time"=1.9142142079681224, "Velocity"=-4.99999999999333}, {"Time"=1.919870458087822, "Velocity"=-4.995067511200252}, {"Time"=1.9255276604175486, "Velocity"=-4.980286918300999}, {"Time"=1.9311846920812694, "Velocity"=-4.95571744866967}, {"Time"=1.9368414152059714, "Velocity"=-4.92145790598746}, {"Time"=1.9424979698836047, "Velocity"=-4.877643862361085}, {"Time"=1.948154953909832, "Velocity"=-4.824442948248025}, {"Time"=1.9538121557145325, "Velocity"=-4.762065523089948}, {"Time"=1.9594690519357183, "Velocity"=-4.690763748968648}, {"Time"=1.9651252996623443, "Velocity"=-4.6108255507610725}, {"Time"=1.9707825265303958, "Velocity"=-4.522542692090294}, {"Time"=1.976439233805907, "Velocity"=-4.42628592603794}, {"Time"=1.982096169164168, "Velocity"=-4.322423047968585}, {"Time"=1.9877531161885007, "Velocity"=-4.2113674555412715}, {"Time"=1.9934097596440727, "Velocity"=-4.093564150396464}, {"Time"=1.999066384653616, "Velocity"=-3.969472657766189}, {"Time"=2.0047232700425024, "Velocity"=-3.839576192421264}, {"Time"=2.0103800975957924, "Velocity"=-3.7043943803591444}, {"Time"=2.016037468304002, "Velocity"=-3.5644457713076045}, {"Time"=2.0216943136137404, "Velocity"=-3.420309078541166}, {"Time"=2.02735127687264, "Velocity"=-3.2725372424230965}, {"Time"=2.033007706221516, "Velocity"=-3.1217307967730683}, {"Time"=2.0386645605970255, "Velocity"=-2.968459438802304}, {"Time"=2.0443218624886894, "Velocity"=-2.813326956495403}, {"Time"=2.0499785612627646, "Velocity"=-2.656974434381646}, {"Time"=2.0556351754128213, "Velocity"=-2.5000047897005144}, {"Time"=2.0612921287868304, "Velocity"=-2.343025725126519}, {"Time"=2.066948951292216, "Velocity"=-2.1866697933857235}, {"Time"=2.0726060344817645, "Velocity"=-2.0315433086293098}, {"Time"=2.0782625112037723, "Velocity"=-1.8782820695613962}, {"Time"=2.0839194703426758, "Velocity"=-1.727461399890248}, {"Time"=2.089576549699353, "Velocity"=-1.5796865967328761}, {"Time"=2.095233002449939, "Velocity"=-1.4355598831706486}, {"Time"=2.1008902395088236, "Velocity"=-1.295614347999071}, {"Time"=2.106546654198525, "Velocity"=-1.1604418971442225}, {"Time"=2.1122035532622414, "Velocity"=-1.030544368061609}, {"Time"=2.117860793765241, "Velocity"=-0.9064388962507246}, {"Time"=2.1235176730524006, "Velocity"=-0.7886306531337383}, {"Time"=2.1291746421594184, "Velocity"=-0.6775747562028543}, {"Time"=2.1348309982289866, "Velocity"=-0.5737222827065941}, {"Time"=2.140487758888143, "Velocity"=-0.47746400611079853}, {"Time"=2.1461447280966754, "Velocity"=-0.38918438898925833}, {"Time"=2.1518019873949377, "Velocity"=-0.3092316555689075}, {"Time"=2.1574587522670696, "Velocity"=-0.23793196833477168}, {"Time"=2.1631154774043555, "Velocity"=-0.17555975540071594}, {"Time"=2.168772601844636, "Velocity"=-0.12235720230915681}, {"Time"=2.1744291901921997, "Velocity"=-0.07854271833129783}, {"Time"=2.18008598338341, "Velocity"=-0.04428265716749067}, {"Time"=2.1857430834919027, "Velocity"=-0.01971291428517812}, {"Time"=2.1913995831337085, "Velocity"=-0.004933630097452645}, {"Time"=2.1970568449331758, "Velocity"=-3.429554397782898e-12}, {"Time"=2.6213203435596424, "Velocity"=0.0}, {"Time"=2.6213203435596424, "Velocity"=0.0}, {"Time"=2.6213203435596424, "Velocity"=0.0}, {"Time"=2.6213203435596424, "Velocity"=0.0}, {"Time"=2.6213203435596424, 
